vi "Write Menue.vi"(8 "error in (no error)":errorcluster, 10 "Menue":refnum<class "MenueItem.lvclass">[](array[class]), 11 "ContexMenue in":refnum<class "ContexMenue.lvclass">) -> (0 "error out":errorcluster, 3 "ContexMenue out":refnum<class "ContexMenue.lvclass">)   [LabVIEW 2016, in "ContexMenue.lvclass"]
uses:
  ContexMenue.lvclass
  MenueItem/MenueItem.lvclass
  System.Windows.Forms
  ContexMenue.lvclass/ContexMenue.ctl
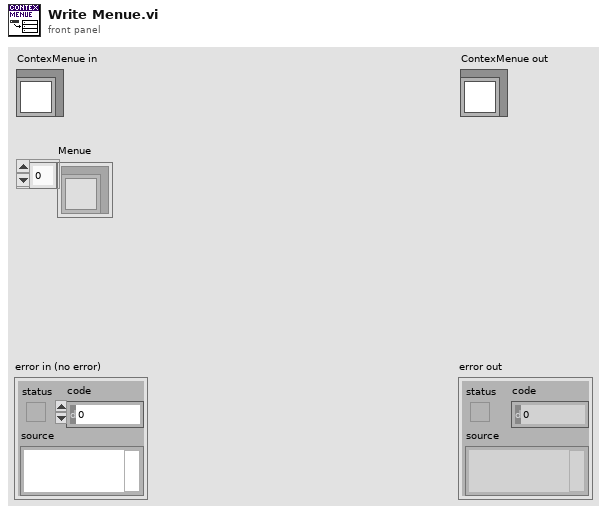
[diagram p1: front panel]
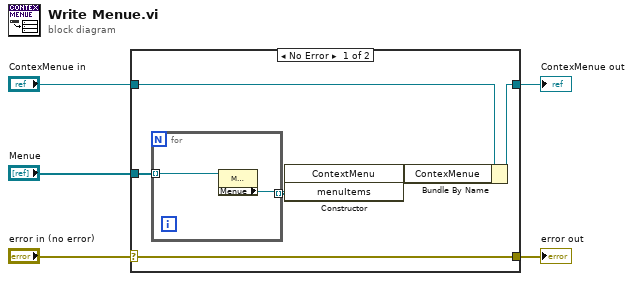
[diagram p0: block diagram]
diagram:
  n1 = case shown="No Error" "error in (no error)" {
    selector: "error in (no error)" -> [w11 w14]
    tunnel: [w11 w14] -> w4
    tunnel: [w10 w15] -> w2
    tunnel: "ContexMenue in" -> [w8 w15]
    tunnel: "Menue" -> [w9 _]
    frame No Error {
      n2 = for {
        tunnel: w9 -> [w13] mode=indexing
        tunnel: [w12] -> w7 mode=indexing
        n3 = property class="MenueItem.lvclass"(reference=w13) -> ("Menue"=w12:refnum<k24>)  [unwired: 1 in, 2 out]
      }
      n4 = constructor class="ContextMenu"("menuItems"=w7) -> (reference out=w6:refnum<k24>)  [unwired: 3 in, 3 out]
      n5 = Bundle By Name(cluster=w8, "ContexMenue"=w6) -> (w10:refnum<class "ContexMenue.lvclass">)
    }
    frame Error {
    }
  }
  "error out" <- w4
  "ContexMenue out" <- w2
